vi "Read ReplayInfo.vi"(8 "error in (no error)":errorcluster, 11 "Game in":refnum<class "Game.lvclass">) -> (0 "error out":errorcluster, 2 "ReplayInfo":T1, 3 "Game out":refnum<class "Game.lvclass">)   [LabVIEW 2023, in "Game.lvclass"]
uses:
  Game.lvclass
  Replay/ReplayInfo.ctl
  Replay/RobotExtraInfo.ctl
  Game.lvclass/Game.ctl
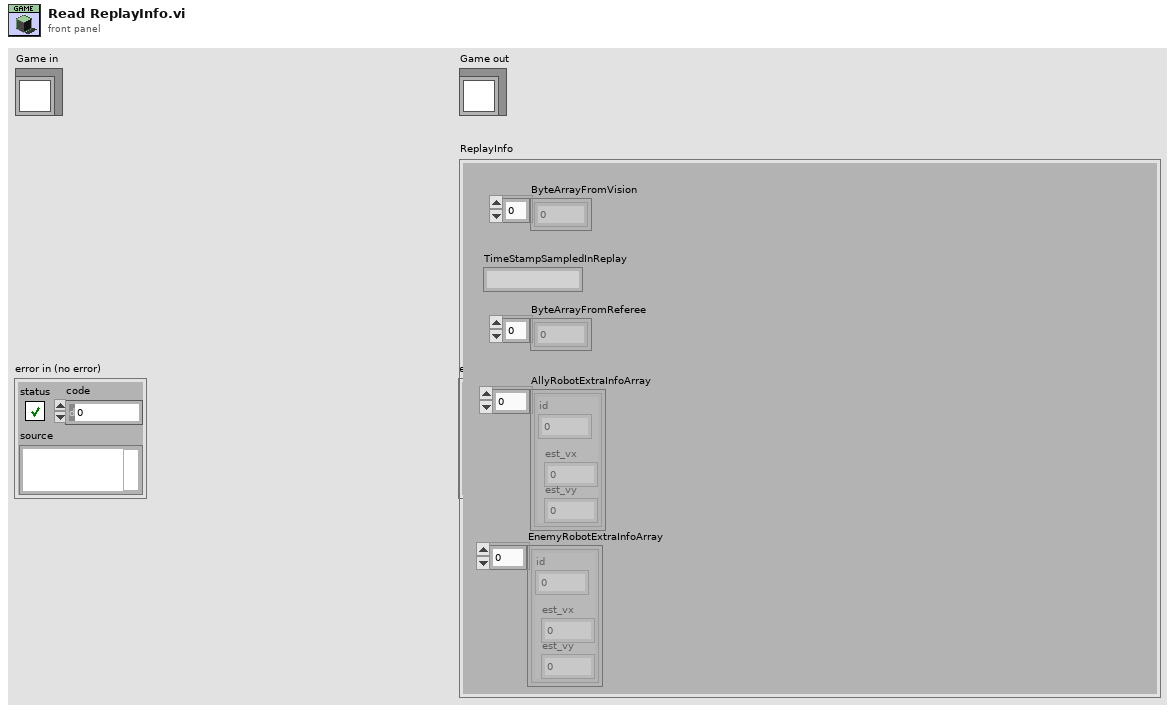
[diagram p1: front panel]
types:
  T1 = typedef "ReplayInfo.ctl" = cluster{"ByteArrayFromVision":u8[], "TimeStampSampledInReplay":string, "ByteArrayFromReferee":u8[], "AllyRobotExtraInfoArray":T2[], "EnemyRobotExtraInfoArray":T2[]}
  T2 = typedef "RobotExtraInfo.ctl" = cluster{"est_vx":dbl, "est_vy":dbl, "id":dbl}
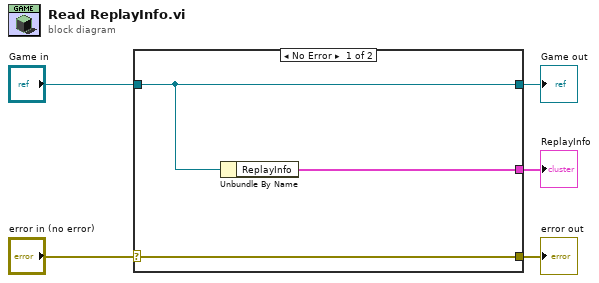
[diagram p0: block diagram]
diagram:
  n1 = case shown="No Error" "error in (no error)" {
    selector: "error in (no error)" -> [w8 w9]
    tunnel: [w8 w9] -> w4
    tunnel: [w7 w10] -> w2
    tunnel: "Game in" -> [w7 w10]
    tunnel: [w6 _] -> w1
    frame No Error {
      n2 = Unbundle By Name(w7) -> ("ReplayInfo"=w6:T1)
    }
    frame Error {
    }
  }
  "error out" <- w4
  "Game out" <- w2
  "ReplayInfo" <- w1
